vi "Finish.vi"(8 "error in (no error)":errorcluster, 11 "Blocker in":refnum<class "Blocker.lvclass">) -> (0 "error out":errorcluster, 3 "Blocker out":refnum<class "Blocker.lvclass">)   [LabVIEW 2013, in "Blocker.lvclass"]
uses:
  Blocker.lvclass
  System/System.lvclass
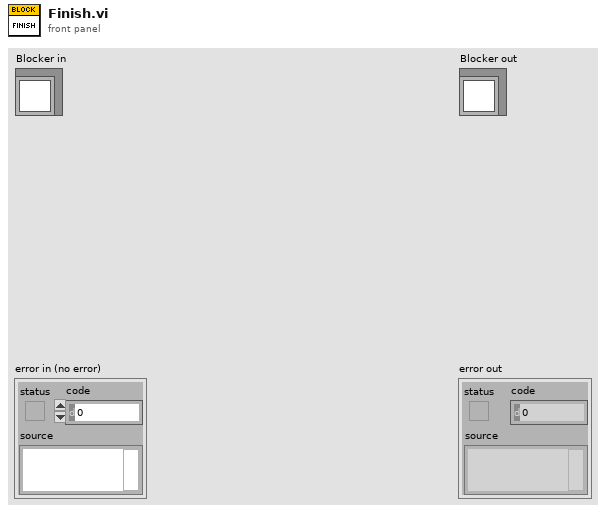
[diagram p1: front panel]
types:
  T1 = typedef "WPI_SolenoidDevRef.ctl" = cluster{"DevStatus":errorcluster, "Solenoid Module":T2, "Forward Solenoid Channel":T3, "Reverse Solenoid Channel":T3}
  T2 = typedef "FPGA_TypedefSolenoidModule.ctl" = enum16{"Solenoid Module 1", "Solenoid Module 2"}
  T3 = typedef "WPI_SolenoidChannel.ctl" = enum8{"Solenoid 1", "Solenoid 2", "Solenoid 3", "Solenoid 4", "Solenoid 5", "Solenoid 6", "Solenoid 7", "Solenoid 8", "Invalid"}
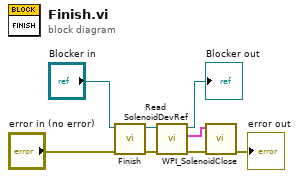
[diagram p0: block diagram]
diagram:
  n1 = call-parent "Finish.vi"("error in (no error)"="error in (no error)", "System in"="Blocker in") -> ("error out"=w3:errorcluster, "System out"=w6:refnum<class "Blocker.lvclass">)  [unwired: 8 in]
  n2 = call-dynamic "Read SolenoidDevRef.vi"("error in (no error)"=w3, "Blocker in"=w6) -> ("error out"=w2:errorcluster, "SolenoidDevRef"=w4:T1, "Blocker out"=→"Blocker out":refnum<class "Blocker.lvclass">)  [unwired: 7 in]
  n3 = call <vilib>:"WPI_SolenoidClose.vi"("error in (no error)"=w2, "SolenoidDevRef"=w4) -> ("error out"=→"error out":errorcluster)  [unwired: 9 in]
